vi "server.vi"() -> ()   [LabVIEW 2014]
panel:
  in  "숫자형":i16 min=0 max=24
  in  "2":bool
  in  "4":bool
  in  "1":bool
  in  "3":bool
  in  "종료취소":bool
  in  "종료":bool
  in  "사용설명서":bool
  out "로그인":bool
  in  "ID":string="ID"
  in  "PW":string="PW"
  in  "명령전달":bool
  in  "address":string="ip address"
  out "참 거짓":string="상태창입니다."
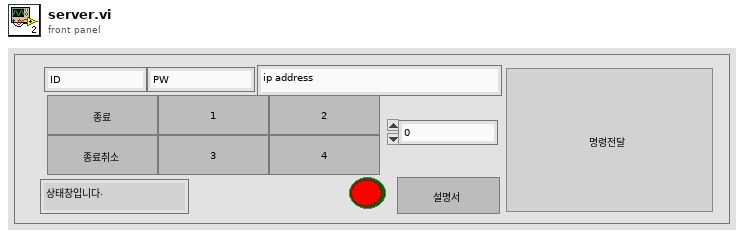
[diagram p1: front panel]
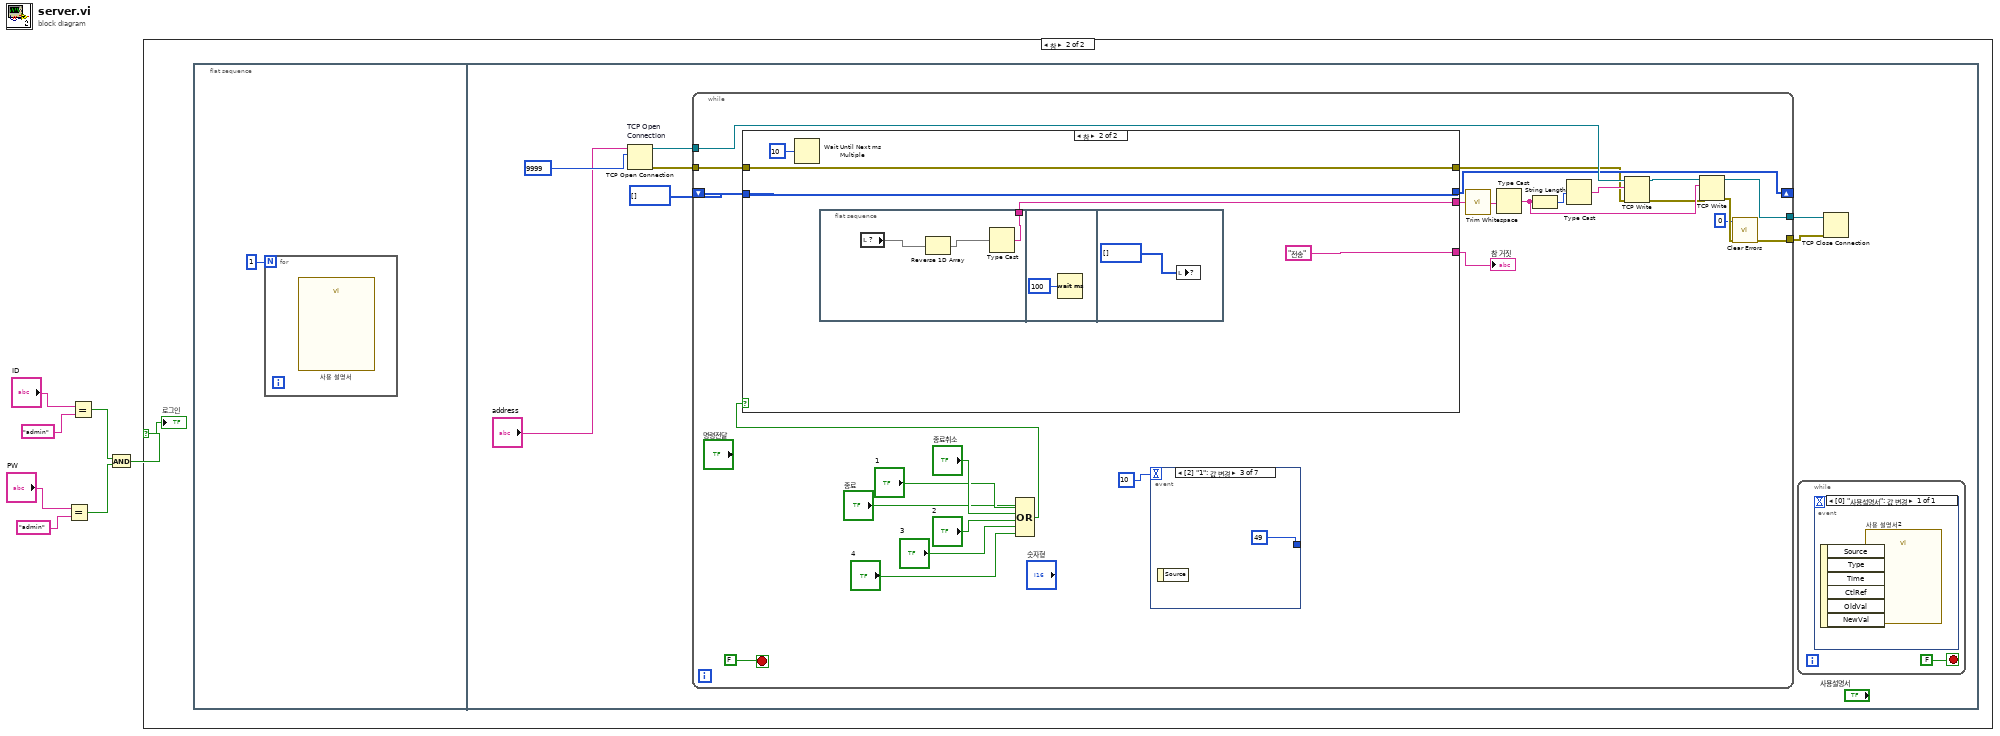
[diagram p0: block diagram]
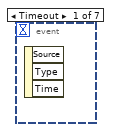
[diagram p3: hidden frame]
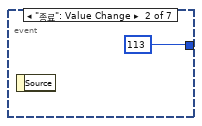
[diagram p4: hidden frame]
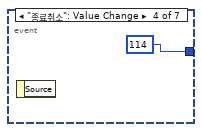
[diagram p5: hidden frame]
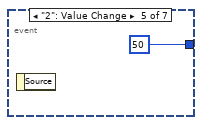
[diagram p6: hidden frame]
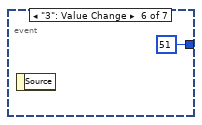
[diagram p7: hidden frame]
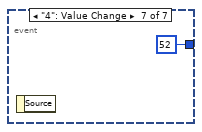
[diagram p8: hidden frame]
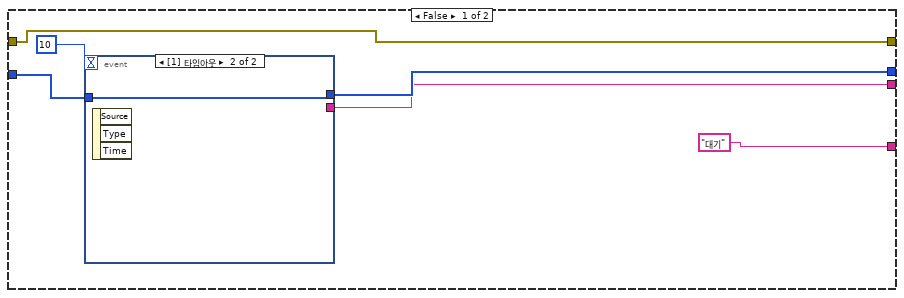
[diagram p9: hidden frame]
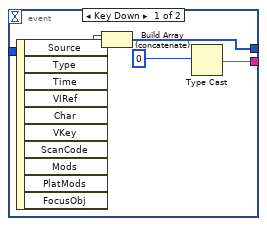
[diagram p10: hidden frame]
diagram:
  n1 = Equal?(x="PW", y="admin") -> (x = y?=w2:bool)
  n2 = Equal?(x="ID", y="admin") -> (x = y?=w3:bool)
  n3 = And(x=w3, y=w2) -> (x .and. y?=w1:bool)
  n4 = case shown="참" w1 {
    selector: w1 -> [_ w8]
    frame False {
    }
    frame True {
      n5 = flat-sequence {
        frame #0 {
          n6 = for {
            N: 1 -> [_]
            n7 = call "사용 설명서"() -> ()  [unwired: 10 in, 2 out]
          }
        }
        frame #1 {
          n8 = TCP Open Connection "TCP Open \nConnection"(address="address", remote port or service name=u16 9999) -> (connection ID=w16:refnum<k5>, error out=w12:errorcluster)  [unwired: 3 in]
          n9 = while {
            tunnel: w16 -> [w41]
            tunnel: [w43] -> w14
            shift-right: [w36] -> _
            shift-left: i16[] [] -> [w42]
            tunnel: w12 -> [w35]
            tunnel: [w28] -> w11
            stop <- FALSE stop-if-true
            n10 = Compound Arithmetic op=OR("종료", "1", "종료취소", "2", "3", "4") -> (w18:bool)
            n11 = case shown="참" w18 {
              tunnel: w42 -> [w55 w66]
              tunnel: [w54 w66] -> w36
              tunnel: [w52 w62] -> w31
              tunnel: w35 -> [w51 w64]
              tunnel: [w51 w64] -> w34
              tunnel: ["대기" "전송"] -> w30
              frame False {
                n12 = event shown="[1] 타임아웃" {
                  selector: _ -> [_ _]
                  dyn-events: _ -> [_ _]
                  timeout: 10 -> [_ _]
                  tunnel: [w59 w61] -> w54
                  tunnel: w55 -> [w60 w61]
                  tunnel: [w57 _] -> w52
                  event Key Down {
                    n13 = event-data() -> ("Char"=w58:i16)  [unwired: 1 in, 9 out]
                    n14 = Build Array (concatenate)(w58, w60) -> (w59:i16[])
                    n15 = Type Cast(x=0) -> (*(type *) &x=w57:string)  [unwired: 1 in]
                  }
                  event Timeout {
                    n16 = event-data() -> ()  [unwired: 1 in, 3 out]
                  }
                }
              }
              frame True {
                n17 = Wait Until Next ms Multiple(millisecond multiple=u32 10) -> ()  [unwired: 1 out]
                n18 = flat-sequence {
                  tunnel: [w68] -> w62
                  frame #0 {
                    n19 = local read item#-1() -> (w69)
                    n20 = Reverse 1D Array(array=w69) -> (reversed array=w67:void[])
                    n21 = Type Cast(x=w67) -> (*(type *) &x=w68:string)  [unwired: 1 in]
                  }
                  frame #1 {
                    n22 = Wait (ms)(milliseconds to wait=u32 100 ("대기 시간(ms)")) -> ()  [unwired: 1 out]
                  }
                  frame #2 {
                    n23 = local write item#-1(i16[] []) -> ()
                  }
                }
              }
            }
            "참 거짓" <- w30
            n24 = event shown="[2] \"1\": 값 변경" {
              selector: _ -> [_ _ _ _ _ _ _]
              dyn-events: _ -> [_ _ _ _ _ _ _]
              timeout: 10 -> [_ _ _ _ _ _ _]
              tunnel: [_ i16 113 i16 49 i16 114 i16 50 i16 51 i16 52] -> _
              event Timeout {
                n25 = event-data() -> ()  [unwired: 1 in, 3 out]
              }
              event "종료": Value Change {
                n26 = event-data() -> ()  [unwired: 1 in, 1 out]
              }
              event "1": Value Change {
                n27 = event-data() -> ()  [unwired: 1 in, 1 out]
              }
              event "종료취소": Value Change {
                n28 = event-data() -> ()  [unwired: 1 in, 1 out]
              }
              event "2": Value Change {
                n29 = event-data() -> ()  [unwired: 1 in, 1 out]
              }
              event "3": Value Change {
                n30 = event-data() -> ()  [unwired: 1 in, 1 out]
              }
              event "4": Value Change {
                n31 = event-data() -> ()  [unwired: 1 in, 1 out]
              }
            }
            n32 = call <vilib>:"Trim Whitespace.vi"("string"=w31) -> ("trimmed string"=w32:string)  [unwired: 1 in]
            n33 = Type Cast(x=w32) -> (*(type *) &x=w37:string)  [unwired: 1 in]
            n34 = String Length(string=w37) -> (length=w38:i32)
            n35 = Type Cast(x=w38) -> (*(type *) &x=w39:string)  [unwired: 1 in]
            n36 = TCP Write(connection ID=w41, data in=w39, error in (no error)=w34) -> (connection ID out=w40:refnum<k5>, error out=w33:errorcluster)  [unwired: 1 in, 1 out]
            n37 = TCP Write(connection ID=w40, data in=w37, error in (no error)=w33) -> (connection ID out=w43:refnum<k5>, error out=w27:errorcluster)  [unwired: 1 in, 1 out]
            n38 = call <vilib>:"Clear Errors.vi"("error in (no error)"=w27, "specific error code to clear (0: all)"=0) -> ("error out"=w28:errorcluster)  [unwired: 4 in, 1 out]
          }
          n39 = while {
            stop <- FALSE stop-if-true
            n40 = event shown="[0] \"사용설명서\": 값 변경" {
              selector: _ -> [_]
              dyn-events: _ -> [_]
              timeout: _ -> [_]
              event "사용설명서": Value Change {
                n41 = event-data() -> ()  [unwired: 1 in, 6 out]
                n42 = call "사용 설명서2"() -> ()  [unwired: 10 in, 2 out]
              }
            }
          }
          n43 = TCP Close Connection(connection ID=w14, error in (no error)=w11) -> ()  [unwired: 1 in, 2 out]
        }
      }
      "로그인" <- w8
    }
  }
